vi "SetDict.vi"(8 "error in (no error)":errorcluster caption="Fehler (Eingang, kein Fehler)", 10 "Dict":variant, 11 "Dictionary (Eingang)":refnum<class "Dictionary.lvclass">) -> (0 "error out":errorcluster caption="Fehler (Ausgang)", 3 "Dictionary (Ausgang)":refnum<class "Dictionary.lvclass">)   [LabVIEW 2013, in "Dictionary.lvclass"]
uses:
  Dictionary.lvclass
  Dictionary.lvclass/Dictionary.ctl
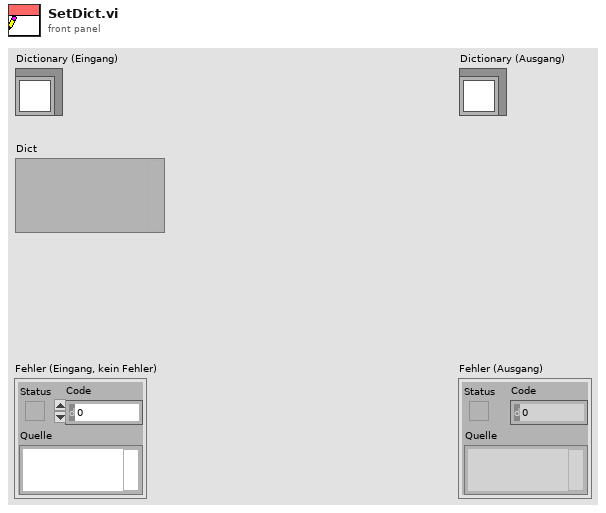
[diagram p1: front panel]
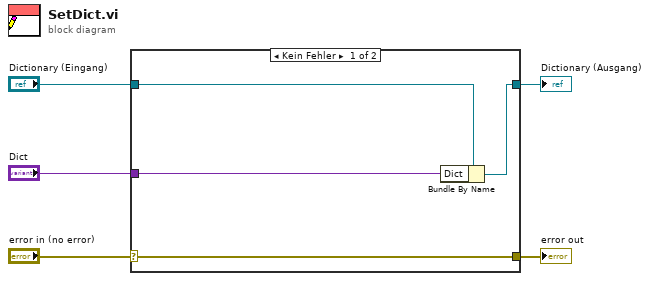
[diagram p0: block diagram]
diagram:
  n1 = case shown="Kein Fehler" "error in (no error)" {
    selector: "error in (no error)" -> [w9 w10]
    tunnel: [w9 w10] -> w4
    tunnel: [w7 w11] -> w2
    tunnel: "Dictionary (Eingang)" -> [w8 w11]
    tunnel: "Dict" -> [w6 _]
    frame No Error {
      n2 = Bundle By Name(cluster=w8, "Dict"=w6) -> (w7:refnum<class "Dictionary.lvclass">)
    }
    frame Error {
    }
  }
  "error out" <- w4
  "Dictionary (Ausgang)" <- w2
